vi "TRIQUI.vi"() -> ()   [LabVIEW 2020]
uses:
  Downloads/TTT2011/Symbol.ctl
panel:
  out "Whos Turn?":string
  in  "Ring 9":u16(ring)
  in  "Ring 8":u16(ring)
  in  "Ring 7":u16(ring)
  in  "Ring 6":u16(ring)
  in  "Ring 5":u16(ring)
  in  "Ring 4":u16(ring)
  in  "Ring 3":u16(ring)
  in  "Ring 2":u16(ring)
  in  "Ring":u16(ring)
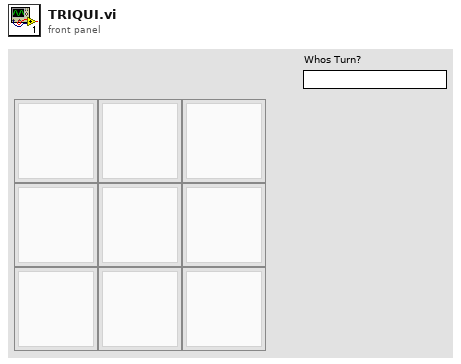
[diagram p1: front panel]
types:
  T1 = typedef "Symbol.ctl" = u16
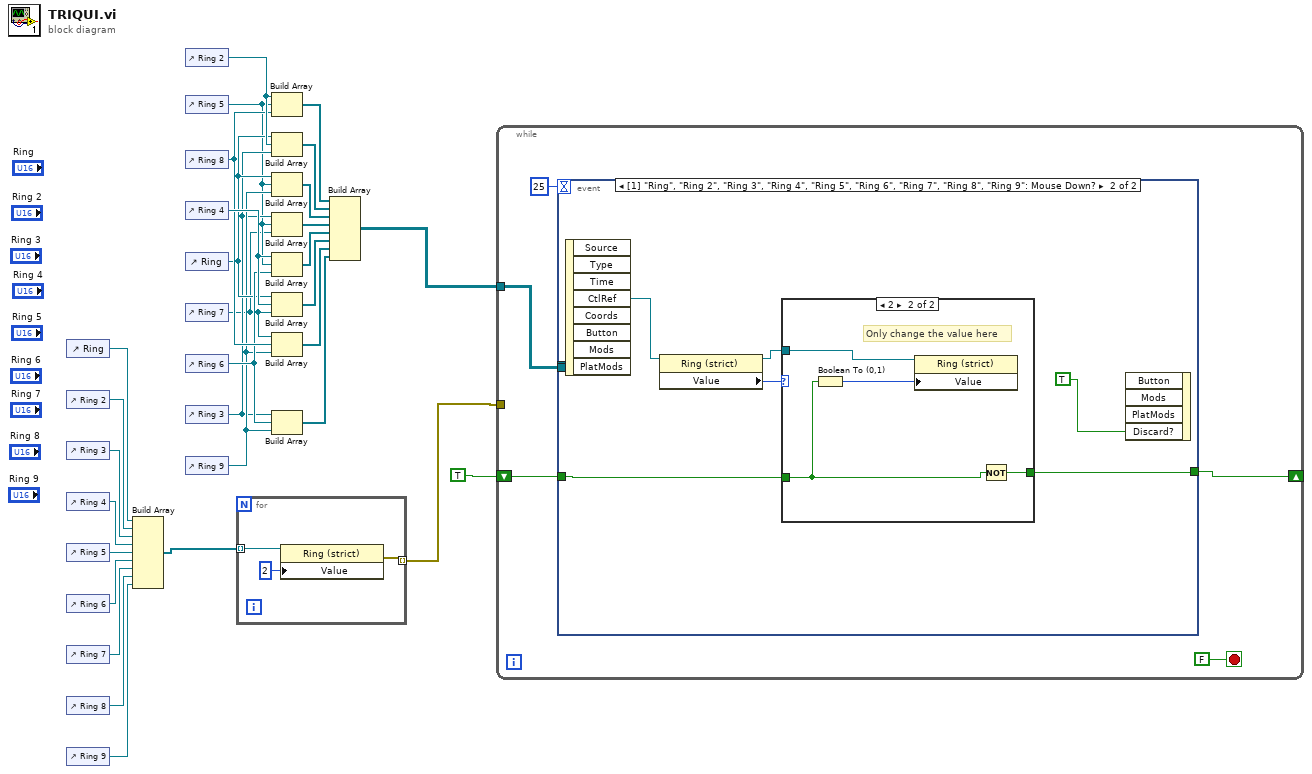
[diagram p0: block diagram]
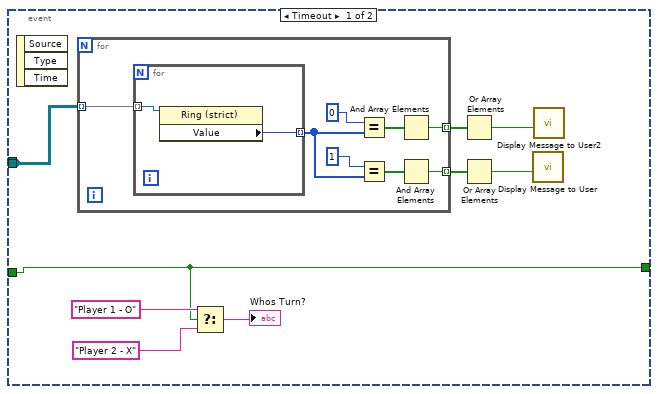
[diagram p2: hidden frame]
diagram:
  n1 = control-ref of="Ring"() -> (w30:refnum<vi>)
  n2 = control-ref of="Ring 2"() -> (w29:refnum<vi>)
  n3 = control-ref of="Ring 3"() -> (w28:refnum<vi>)
  n4 = control-ref of="Ring 4"() -> (w27:refnum<vi>)
  n5 = control-ref of="Ring 5"() -> (w26:refnum<vi>)
  n6 = control-ref of="Ring 6"() -> (w4:refnum<vi>)
  n7 = control-ref of="Ring 7"() -> (w3:refnum<vi>)
  n8 = control-ref of="Ring 8"() -> (w2:refnum<vi>)
  n9 = control-ref of="Ring 9"() -> (w1:refnum<vi>)
  n10 = Build Array(w30, w29, w28, w27, w26, w4, w3, w2, w1) -> (w25:refnum<vi>[])
  n11 = control-ref of="Ring 2"() -> (w23:refnum<vi>)
  n12 = control-ref of="Ring 5"() -> (w17:refnum<vi>)
  n13 = control-ref of="Ring 8"() -> (w22:refnum<vi>)
  n14 = control-ref of="Ring 4"() -> (w24:refnum<vi>)
  n15 = control-ref of="Ring"() -> (w20:refnum<vi>)
  n16 = control-ref of="Ring 7"() -> (w16:refnum<vi>)
  n17 = control-ref of="Ring 6"() -> (w21:refnum<vi>)
  n18 = control-ref of="Ring 3"() -> (w18:refnum<vi>)
  n19 = control-ref of="Ring 9"() -> (w19:refnum<vi>)
  n20 = for {
    tunnel: w25 -> [w33] mode=indexing
    tunnel: [w31] -> w5 mode=indexing
    n21 = property class="Ring (strict)"(reference=w33, "Value"=u16 2) -> (error out=w31:errorcluster)  [unwired: 1 in, 1 out]
  }
  n22 = Build Array(w23, w17, w22) -> (w15:refnum<vi>[])
  n23 = Build Array(w20, w23, w18) -> (w14:refnum<vi>[])
  n24 = Build Array(w20, w17, w19) -> (w13:refnum<vi>[])
  n25 = Build Array(w18, w17, w16) -> (w12:refnum<vi>[])
  n26 = Build Array(w24, w17, w21) -> (w11:refnum<vi>[])
  n27 = Build Array(w20, w24, w16) -> (w10:refnum<vi>[])
  n28 = Build Array(w16, w22, w19) -> (w9:refnum<vi>[])
  n29 = Build Array(w18, w21, w19) -> (w8:refnum<vi>[])
  n30 = Build Array(w15, w14, w13, w12, w11, w10, w9, w8) -> (w7:refnum<vi>[][])
  n31 = while {
    tunnel: w7 -> [w38]
    shift-right: [w36] -> _
    shift-left: TRUE -> [w37]
    tunnel: w5 -> [_]
    stop <- FALSE stop-if-true
    n32 = event shown="[1] \"Ring\", \"Ring 2\", \"Ring 3\", \"Ring 4\", \"Ring 5\", \"Ring 6\", \"Ring 7\", \"Ring 8\", \"Ring 9\": Mouse Down?" {
      selector: _ -> [_ _]
      dyn-events: _ -> [_ _]
      timeout: 25 -> [_ _]
      tunnel: [w39 _] -> _
      tunnel: w38 -> [w39 _]
      tunnel: w37 -> [w40 w60]
      tunnel: [w40 w59] -> w36
      event Timeout {
        n33 = event-data() -> ()  [unwired: 1 in, 3 out]
        n34 = for {
          tunnel: [w50] -> w43 mode=indexing
          tunnel: [w49] -> w44 mode=indexing
          tunnel: w39 -> [w48] mode=indexing
          n35 = for {
            tunnel: [w57] -> w53 mode=indexing
            tunnel: w48 -> [w56] mode=indexing
            n36 = property class="Ring (strict)"(reference=w56) -> ("Value"=w57:T1)  [unwired: 1 in, 2 out]
          }
          n37 = Equal?(x=T1 0 ("Value"), y=w53) -> (x = y?=w52:bool[])
          n38 = Equal?(x=T1 1 ("Value"), y=w53) -> (x = y?=w51:bool[])
          n39 = And Array Elements(Boolean array=w52) -> (logical AND=w49:bool)
          n40 = And Array Elements(Boolean array=w51) -> (logical AND=w50:bool)
        }
        n41 = Select(t="Player 1 - O", s=w40, f="Player 2 - X") -> (s? t:f=→"Whos Turn?":string)
        n42 = Or Array Elements(Boolean array=w44) -> (logical OR=w42:bool)
        n43 = Or Array Elements(Boolean array=w43) -> (logical OR=w41:bool)
        n44 = call "Display Message to User"("Enable"=w41) -> ()  [unwired: 9 in, 2 out]
        n45 = call "Display Message to User2"("Enable"=w42) -> ()  [unwired: 9 in, 2 out]
      }
      event "Ring", "Ring 2", "Ring 3", "Ring 4", "Ring 5", "Ring 6", "Ring 7", "Ring 8", "Ring 9": Mouse Down? {
        n46 = event-data() -> ("CtlRef"=w58:refnum<vi>)  [unwired: 1 in, 7 out]
        n47 = property class="Ring (strict)"(reference=w58) -> (reference out=w62:refnum<vi>, "Value"=w63:T1)  [unwired: 1 in, 1 out]
        n48 = case shown="2" w63 {
          tunnel: [w64 w68] -> w59
          tunnel: w62 -> [_ w67]
          tunnel: w60 -> [w64 w65]
          frame Default {
            # "DO not touch the values here"
          }
          frame 2 {
            # "Only change the value here"
            n49 = Boolean To (0,1)(Boolean=w65) -> (0, 1=w66:i16)
            n50 = property class="Ring (strict)"(reference=w67, "Value"=w66) -> ()  [unwired: 1 in, 2 out]
            n51 = Not(x=w65) -> (.not. x?=w68:bool)
          }
        }
        n52 = event-data("Discard?"=TRUE) -> ()  [unwired: 4 in, 1 out]
      }
    }
  }
